vi "general query.vi"() -> ()   [LabVIEW 2009]
panel:
  out "VISA resource name out":refnum<visa-resource-name>
  out "error out":errorcluster
  in  "error in (no error)":errorcluster
  in  "VISA resource name":refnum<visa-resource-name>="GPIB0::21::INSTR"
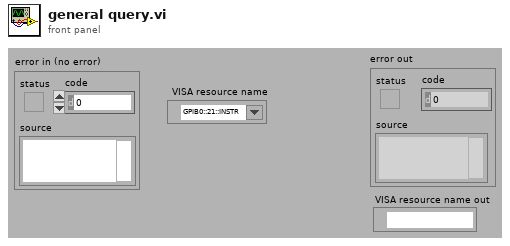
[diagram p1: front panel]
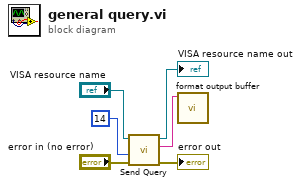
[diagram p0: block diagram]
diagram:
  n1 = call "Send Query.vi"("error in (no error)"="error in (no error)", "Bytes Count"=14, "VISA resource name"="VISA resource name") -> ("error out"=→"error out":errorcluster, "read buffer"=w1:string, "VISA resource name out"=→"VISA resource name out":refnum<visa-resource-name>)  [unwired: 6 in]
  n2 = call "format output buffer.vi"("read buffer"=w1) -> ()  [unwired: 11 in]
